vi "Vision Aim Gyro.vi"(11 "abort":bool) -> (0 "ARM GOOD":bool, 1 "WHEELS GOOD":bool, 2 "Vision In Range?":bool, 3 "Gyro":dbl format="%.2f")   [LabVIEW 2015]
uses:
  <vilib>/addons/control/pid/pid.llb/PID Control Input Filter (DBL).vi
  Code/Robot Global Data.vi
  <vilib>/addons/control/pid/NI_PID_pid.lvlib
panel:
  in  "Vision Tolerance":dbl=0.05
  in  "Turn PID gains":T1={"proportional gain (Kc)"=0.008, "integral time (Ti, min)"=0.0, "derivative time (Td, min)"=0.0013}
  in  "Reset gyro":bool
  in  "F gain":dbl=0.5
  out "Angel out":dbl
  out "Output":dbl
  out "Angle To Turn":dbl
  # "Outputs"
  # "Turning Gains"
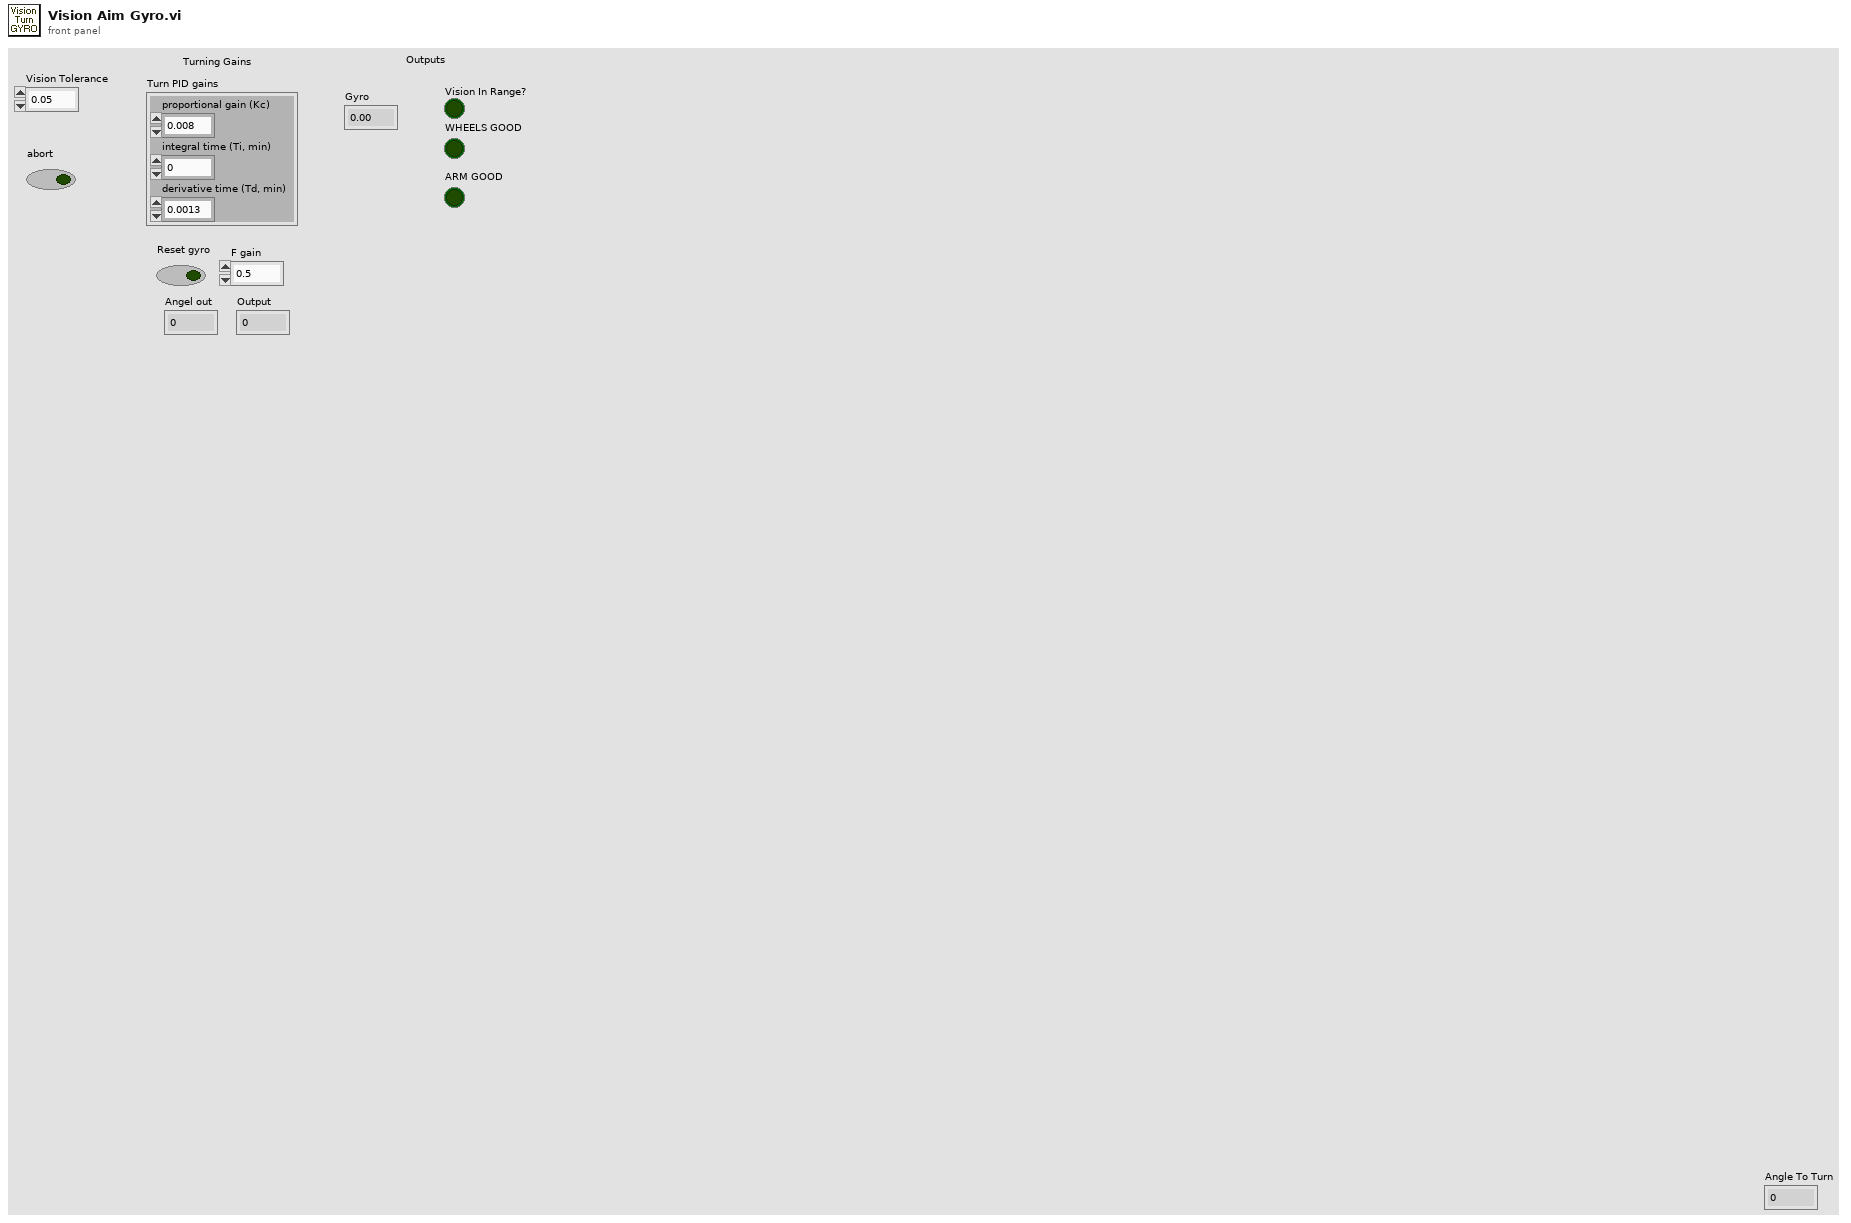
[diagram p1: front panel]
types:
  T1 = cluster{"proportional gain (Kc)":dbl, "integral time (Ti, min)":dbl, "derivative time (Td, min)":dbl}
  T2 = enum16{"Init", "Get Angle", "Turn Angle ", "Shoot?", "Stop"}
  T3 = typedef "WPI_GyroDevRef.ctl" = cluster{"DevStatus":errorcluster, "Analog Channel":T4, "Offset":dbl, "Gain (VoltsPerDegree/Second)":dbl, "Gyro Type":enum16{"Analog", "XRS450"}, "Handle":i32, "SPI Bus":T5, "Device Found":bool, "Sample Rate":dbl, "Calibrate On Open":bool}
  T4 = typedef "FPGA_AIChannel.ctl" = enum8{"AI 0", "AI 1", "AI 2", "AI 3", "AI MXP 0", "AI MXP 1", "AI MXP 2", "AI MXP 3", "Invalid"}
  T5 = typedef "spi_bus.ctl" = enum16{"SPI On-Board, CS0", "SPI On-Board, CS1", "SPI On-Board, CS2", "SPI On-Board, CS3", "SPI MXP", "Invalid"}
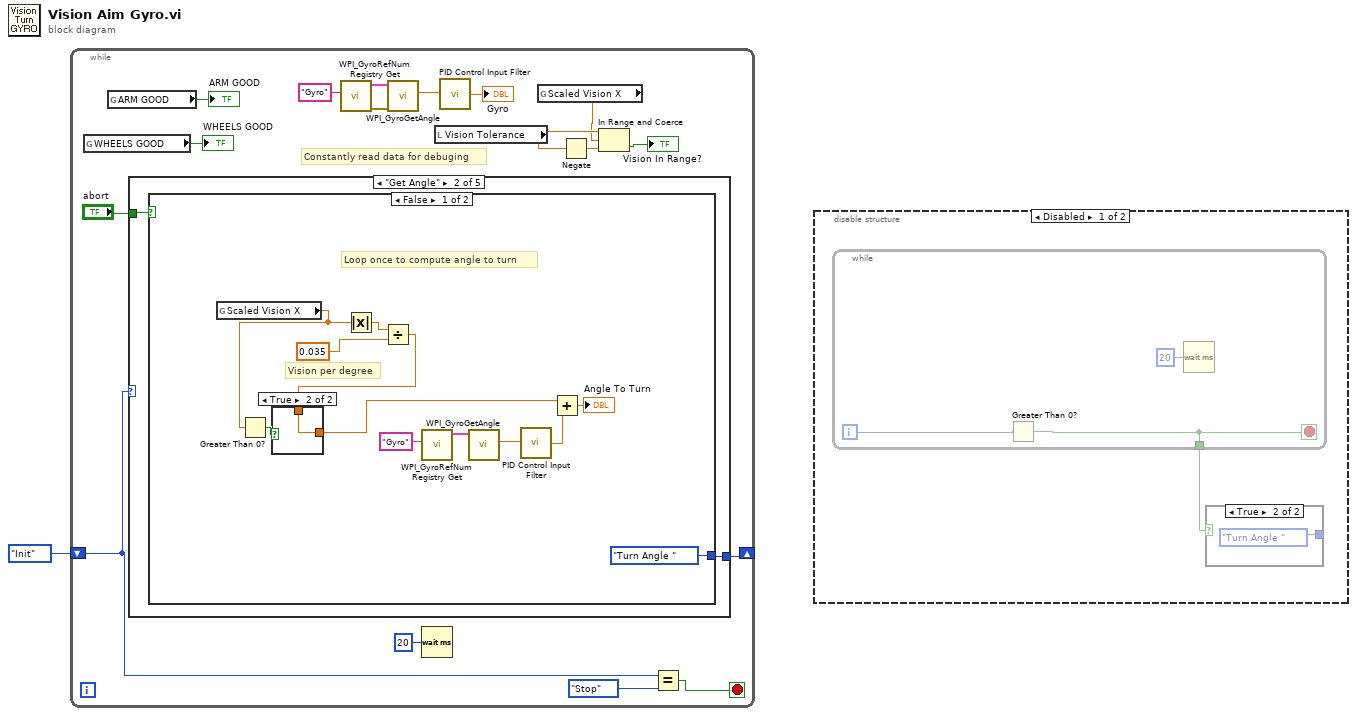
[diagram p0: block diagram]
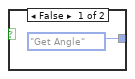
[diagram p2: hidden frame]
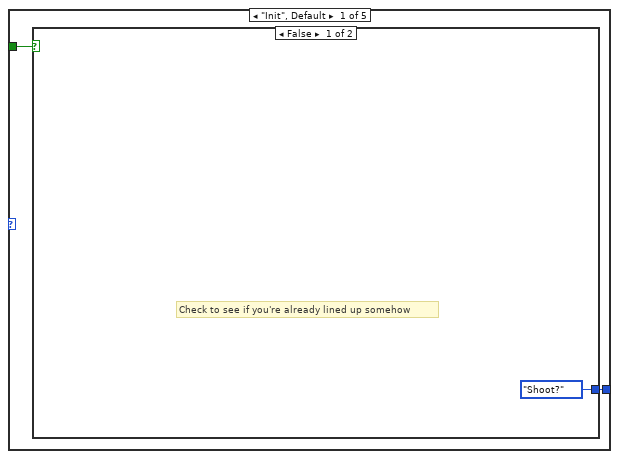
[diagram p4: hidden frame]
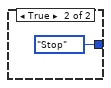
[diagram p5: hidden frame]
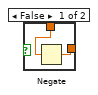
[diagram p6: hidden frame]
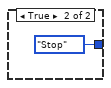
[diagram p7: hidden frame]
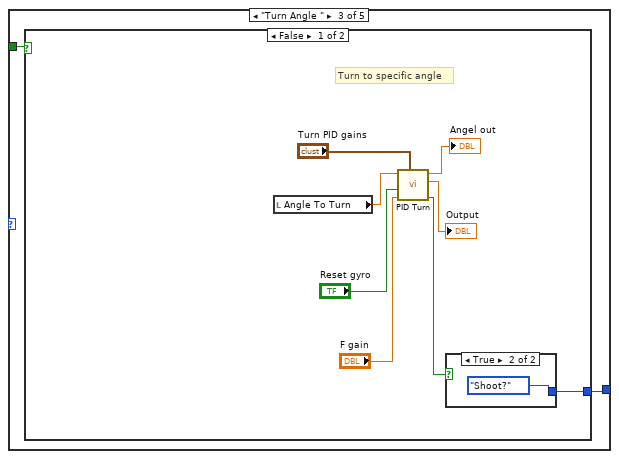
[diagram p8: hidden frame]
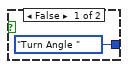
[diagram p9: hidden frame]
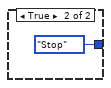
[diagram p10: hidden frame]
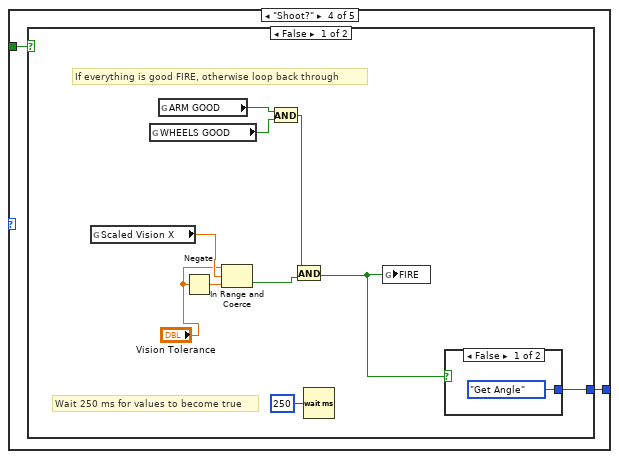
[diagram p11: hidden frame]
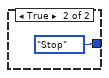
[diagram p12: hidden frame]
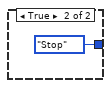
[diagram p13: hidden frame]
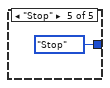
[diagram p14: hidden frame]
diagram:
  n1 = while {
    shift-right: [w17] -> _
    shift-left: T2."Init" -> [w15]
    stop <- w16 stop-if-true
    # "Constantly read data for debuging"
    n2 = global read "Robot Global Data.vi" "WHEELS GOOD"() -> (→"WHEELS GOOD":bool)
    n3 = global read "Robot Global Data.vi" "ARM GOOD"() -> (→"ARM GOOD":bool)
    n4 = case shown="\"Get Angle\"" w15 {
      tunnel: "abort" -> [w20 w23 w42 w54 _]
      tunnel: [w19 w24 w41 w55 T2."Stop"] -> w17
      frame "Init", Default {
        n5 = case shown="False" w20 {
          tunnel: [T2."Shoot?" T2."Stop"] -> w19
          frame False {
            # "Check to see if you're already lined up somehow"
          }
          frame True {
          }
        }
      }
      frame "Get Angle" {
        n6 = case shown="False" w23 {
          tunnel: [T2."Turn Angle " T2."Stop"] -> w24
          frame False {
            # "Loop once to compute angle to turn"
            # "Vision per degree"
            n7 = global read "Robot Global Data.vi" "Scaled Vision X"() -> (w32:dbl)
            n8 = Greater Than 0?(x=w32) -> (x > 0?=w28:bool)
            n9 = Absolute Value(x=w32) -> (abs(x)=w26:dbl)
            n10 = Divide(x=w26, y=0.035) -> (x/y=w29:dbl)
            n11 = case shown="True" w28 {
              tunnel: [w38 w39] -> w30
              tunnel: w29 -> [w37 w39]
              frame False {
                n12 = Negate(x=w37) -> (-x=w38:dbl)
              }
              frame True {
              }
            }
            n13 = call <vilib>:"WPI_GyroRefNum Registry Get.vi"("refnum name"="Gyro") -> ("GyroDevRef"=w34:T3)  [unwired: 9 in, 1 out]
            n14 = call <vilib>:"WPI_GyroGetAngle.vi"("GyroDevRef"=w34) -> ("Angle"=w35:dbl)  [unwired: 6 in, 4 out]
            n15 = call-poly <vilib>:"PID Control Input Filter.vi"("input"=w35) -> ("output"=w36:dbl)  [unwired: 4 in]
            n16 = Add(x=w30, y=w36) -> (x+y=→"Angle To Turn":dbl)
          }
          frame True {
          }
        }
      }
      frame "Turn Angle " {
        n17 = case shown="False" w42 {
          tunnel: [w50 T2."Stop"] -> w41
          frame False {
            # "Turn to specific angle"
            n18 = local read "Angle To Turn"() -> (w49:dbl)
            n19 = call "PID Turn.vi"("PID gains"="Turn PID gains", "F gain"="F gain", "Reset gyro"="Reset gyro", "Setpoint"=w49) -> ("Done"=w43:bool, "Output"=→"Output":dbl, "Angel out"=→"Angel out":dbl)  [unwired: 5 in]
            n20 = case shown="True" w43 {
              tunnel: [T2."Turn Angle " T2."Shoot?"] -> w50
              frame False {
              }
              frame True {
              }
            }
          }
          frame True {
          }
        }
      }
      frame "Shoot?" {
        n21 = case shown="False" w54 {
          tunnel: [w65 T2."Stop"] -> w55
          frame False {
            # "Wait 250 ms for values to become true"
            # "If everything is good FIRE, otherwise loop back through"
            n22 = global read "Robot Global Data.vi" "Scaled Vision X"() -> (w60:dbl)
            n23 = global read "Robot Global Data.vi" "WHEELS GOOD"() -> (w61:bool)
            n24 = global read "Robot Global Data.vi" "ARM GOOD"() -> (w62:bool)
            n25 = Negate(x="Vision Tolerance") -> (-x=w58:dbl)
            n26 = In Range and Coerce(upper limit="Vision Tolerance", x=w60, lower limit=w58) -> (In Range?=w63:bool)  [unwired: 1 out]
            n27 = And(x=w62, y=w61) -> (x .and. y?=w64:bool)
            n28 = And(x=w64, y=w63) -> (x .and. y?=w56:bool)
            n29 = Wait (ms)(milliseconds to wait=u32 250) -> ()  [unwired: 1 out]
            n30 = global write "Robot Global Data.vi" "FIRE"(w56) -> ()
            n31 = case shown="False" w56 {
              tunnel: [T2."Get Angle" T2."Stop"] -> w65
              frame False {
              }
              frame True {
              }
            }
          }
          frame True {
          }
        }
      }
      frame "Stop" {
      }
    }
    n32 = call <vilib>:"WPI_GyroRefNum Registry Get.vi"("refnum name"="Gyro") -> ("error out"=w5:errorcluster, "GyroDevRef"=w4:T3)  [unwired: 9 in]
    n33 = call <vilib>:"WPI_GyroGetAngle.vi"("error in"=w5, "GyroDevRef"=w4) -> ("Angle"=w3:dbl)  [unwired: 5 in, 4 out]
    n34 = Wait (ms)(milliseconds to wait=u32 20) -> ()  [unwired: 1 out]
    n35 = local read "Vision Tolerance"() -> (w12:dbl)
    n36 = call-poly <vilib>:"PID Control Input Filter.vi"("input"=w3) -> ("output"=→"Gyro":dbl)  [unwired: 4 in]
    n37 = global read "Robot Global Data.vi" "Scaled Vision X"() -> (w10:dbl)
    n38 = Negate(x=w12) -> (-x=w11:dbl)
    n39 = In Range and Coerce(upper limit=w12, x=w10, lower limit=w11) -> (In Range?=→"Vision In Range?":bool)  [unwired: 1 out]
    n40 = Equal?(x=w15, y=T2."Stop") -> (x = y?=w16:bool)
  }
  n41 = disable-structure shown="Disabled" {
    frame Disabled {
      n42 = while {
        tunnel: [w75] -> w70
        i -> [w74]
        stop <- w75 stop-if-true
        n43 = Greater Than 0?(x=w74) -> (x > 0?=w75:bool)
        n44 = Wait (ms)(milliseconds to wait=u32 20) -> ()  [unwired: 1 out]
      }
      n45 = case shown="True" w70 {
        tunnel: [T2."Get Angle" T2."Turn Angle "] -> _
        frame False {
        }
        frame True {
        }
      }
    }
    frame Enabled {
    }
  }
